vi "DataLogger.ResetAlarms.vi"(8 "error in (no error)":errorcluster, 11 "i ref in":refnum<vi>) -> (0 "error out":errorcluster, 3 "i ref out":refnum<vi>)   [LabVIEW 2014, in "DataLogger.lvlib"]
uses:
  DataLogger.lvlib
  CSlibraries-extern/DimLVEvent/LVDimInterface/LVDimInterface.lvlib
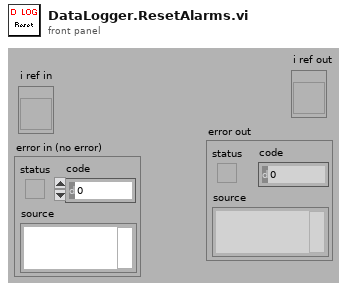
[diagram p1: front panel]
types:
  T1 = enum16{"open", "replace", "create", "open or create", "replace or create", "replace or create with confirmation"}
  T2 = typedef "DataLogger.lvlib/DataLogger.i attribute.ctl" = cluster{"Service Names":string[], "Path":string[], "Service Alarm Index":i32[], "Service Alarm Limit1":dbl[], "Service Alarm Limit2":dbl[], "Service Alarm Indicator":bool[], "alarmID":i32, "pathID":i32, "SoundDeviceID":i32, "SoundFile":string, "SoundID":i32, "SoundFileID":i32}
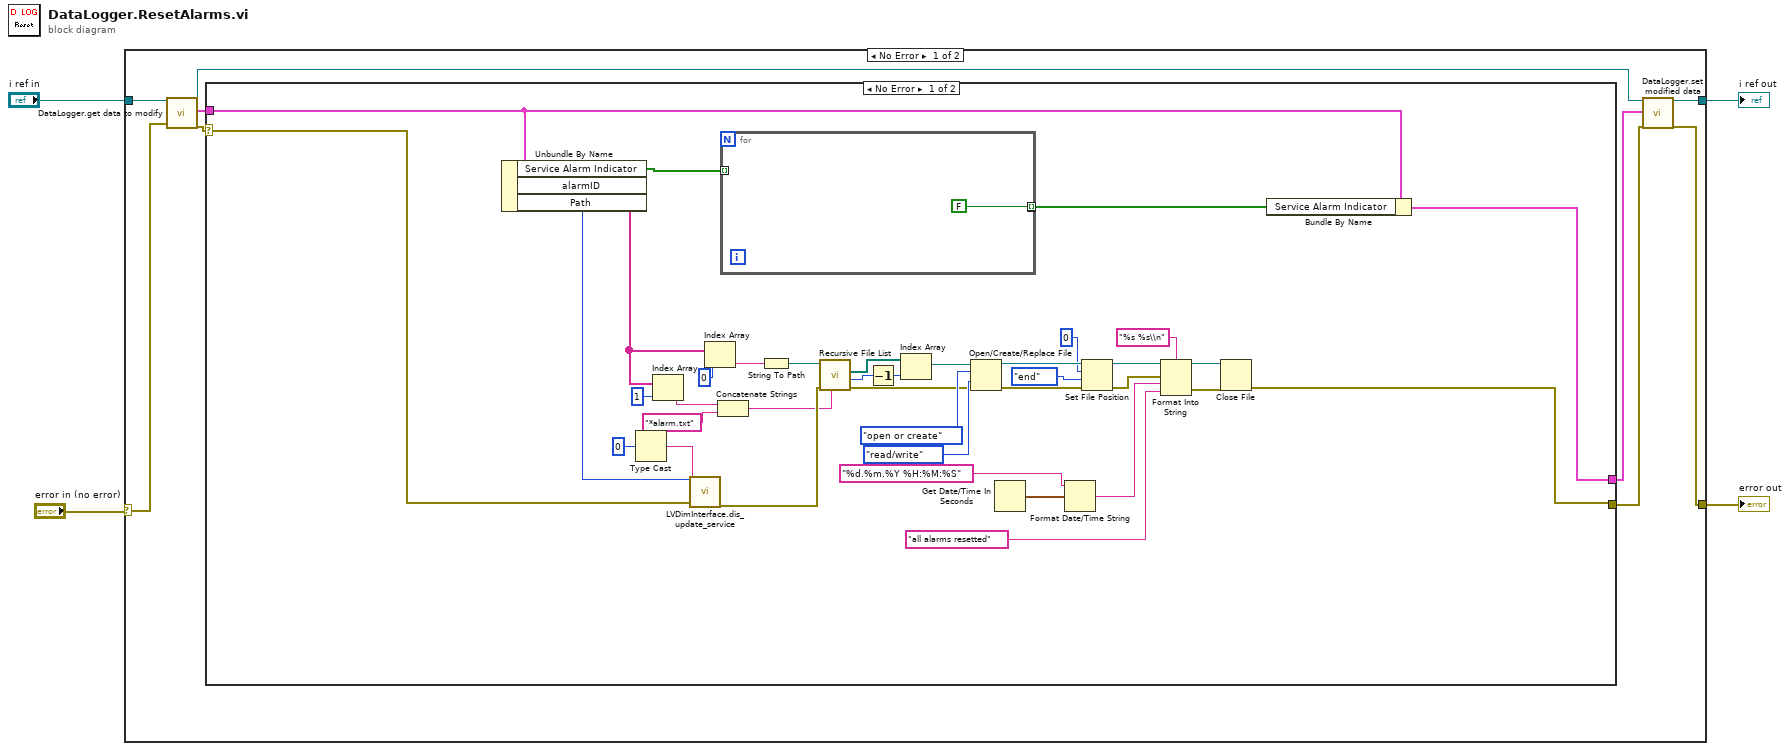
[diagram p0: block diagram]
diagram:
  n1 = case shown="No Error" "error in (no error)" {
    selector: "error in (no error)" -> [w12 w55]
    tunnel: "i ref in" -> [w13 w56]
    tunnel: [w8 w56] -> w2
    tunnel: [w6 w55] -> w1
    frame No Error {
      n2 = call "DataLogger.get data to modify.vi"("i ref in"=w13, "error in (no error)"=w12) -> ("i ref out"=w9:refnum<vi>, "i attribute"=w11:T2, "error out"=w10:errorcluster)  [unwired: 14 in, 1 out]
      n3 = case shown="No Error" w10 {
        selector: w10 -> [w45 w54]
        tunnel: w11 -> [w48 w53]
        tunnel: [w22 w54] -> w7
        tunnel: [w51 w53] -> w5
        frame No Error {
          n4 = Unbundle By Name(w48) -> ("Service Alarm Indicator"=w50:bool[], "alarmID"=w44:i32, "Path"=w18:string[])
          n5 = Type Cast(x=0) -> (*(type *) &x=w46:string)  [unwired: 1 in]
          n6 = Index Array(array=w18, index=1) -> (element=w16:string)
          n7 = call "LVDimInterface.dis_update_service.vi"("my_serviceID"=w44, "data"=w46, "error in (no error)"=w45) -> ("error out"=w28:errorcluster)  [unwired: 14 in, 2 out]
          n8 = Index Array(array=w18, index=0 ("length")) -> (element=w43:string)
          n9 = Concatenate Strings(w16, "*alarm.txt" ("pattern")) -> (w14:string)
          n10 = for {
            tunnel: w50 -> [_] mode=indexing
            tunnel: [w52] -> _ mode=indexing
            tunnel: [w52] -> w49 mode=indexing
            w52 = FALSE
          }
          n11 = String To Path(string=w43) -> (path=w41:path)
          n12 = call <vilib>:"Recursive File List.vi"("pattern"=w14, "error in (no error)"=w28, "Folder Path"=w41) -> ("error out"=w27:errorcluster, "Number of Files"=w20:i32, "All Files in Dir"=w29:path[])  [unwired: 4 in, 2 out]
          n13 = Decrement(x=w20) -> (x-1=w19:i32)
          n14 = Index Array(array=w29, index=w19) -> (element=w21:path)
          n15 = Open/Create/Replace File(file path (use dialog)=w21, error in=w27, operation (0:open)=T1."open or create", access (0:read/write)=enum16{"read/write", "read-only", "write-only"}."read/write") -> (refnum out=w35:refnum<file>, error out=w34:errorcluster)  [unwired: 2 in, 1 out]
          n16 = Get Date/Time In Seconds() -> (seconds since 1Jan1904=w24:timestamp)
          n17 = Format Date/Time String(time format string (%c)="%d.%m.%Y %H:%M:%S", seconds (now)=w24) -> (date/time string=w26:string)  [unwired: 1 in]
          n18 = Set File Position(offset (in bytes) (0)=i64 0, refnum=w35, from (0:start)=enum16{"start", "end", "current"}."end", error in=w34) -> (refnum out=w32:refnum<file>, error out=w33:errorcluster)
          n19 = Format Into String(format string="%s %s\\n", initial string=w32, error in=w33, w26, "all alarms resetted" ("input 2")) -> (resulting string=w38:refnum<file>, error out=w39:errorcluster)
          n20 = Close File(refnum=w38, error in=w39) -> (error out=w22:errorcluster)  [unwired: 1 out]
          n21 = Bundle By Name(cluster=w48, "Service Alarm Indicator"=w49) -> (w51:T2)
        }
        frame Error {
        }
      }
      n22 = call "DataLogger.set modified data.vi"("i ref in"=w9, "i attribute"=w5, "error in (no error)"=w7) -> ("i ref out"=w8:refnum<vi>, "error out"=w6:errorcluster)  [unwired: 15 in]
    }
    frame Error {
    }
  }
  "error out" <- w1
  "i ref out" <- w2
